vi "nearCamReConnect.vi"(2 "error in":errorcluster, 3 "Session In":T1) -> (0 "错误输出":errorcluster, 1 "IMAQdx Session Out":T1)   [LabVIEW 2018]
uses:
  <vilib>/userdefined/High Color/IMAQdx.ctl
  <vilib>/vision/driver/NI_Vision_Acquisition_Software.lvlib
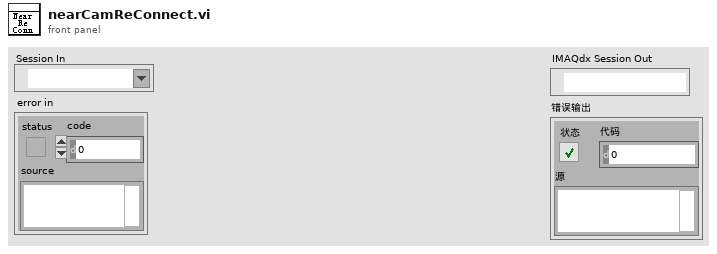
[diagram p1: front panel]
types:
  T1 = typedef "IMAQdx.ctl" = refnum<k21>
  T2 = typedef "IMAQ Image.ctl" = refnum<image>
  T3 = cluster{"示波器":cluster{"Channel (0:Channel 1)":enum16{"Channel 1", "Channel 2", "Channel 3", "Channel 4"}, "电压范围":dbl, "触发电压":dbl, "时间范围":dbl, " 示波器VISA":refnum<visa-resource-name>, "时间范围 标签":u64, "电压范围 标签":u64, "触发电压 标签":u64, "输入阻抗/Ω":u64}, "光谱仪":cluster{"SpecDataReference":refnum<queue>, "grating center":dbl, "Exposure Time (s)":dbl, "是否进行详细设置":bool, " 开始通信检查":bool, "通信成功？":bool, "波长":dbl}, " 近场相机":cluster{"曝光时间/us":dbl, "模拟增益":i32, "控制套接字":i32, "IP 地址":string, " 采集套接字":i32, "  版本号":i32, "ImageData":T2, "  增益最大":i32, "  增益最小":i32, " 曝光最大":i32, " 曝光最小":i32, " 帧速":i32, " 同步切换":i32, "  曝光缩放":i32, "Camera Source":refnum<k21>, "近场X范围":dbl, "近场Y范围":dbl, "单个像元大小/um":dbl, "相机距离原点位置":dbl[], "是否测量发散角":bool, "光束类型(发散T)":bool, "聚焦透镜焦距mm":dbl}, " 偏振仪":cluster{"电压范围":u64, "触发电压":u64, "时间范围":u64, "波长范围":enum16{"可见光 400-700nm", "近红外 700-1100nm"}, "可见光偏振测量仪VISA":refnum<visa-resource-name>, "近红外偏振测量仪VISA":refnum<visa-resource-name>}, " 功率计":cluster{"通道":enum16{"Channel 1", "Channel 2"}, "工作波长":u32, "单位":u64, "时间范围":u64, "IP地址":string, "端口":u32, "是否需要散射片":bool}, "能量计":cluster{"通道":enum16{"Channel 1", "Channel 2"}, "工作波长":u32, "单位":u64, "时间范围":u64, "IP地址":string, "端口":u32, "能量计量程":enum16{"200uJ", "20uJ", "2uJ", "200nJ"}}, "电机":cluster{"Channel (0:Channel 1)":enum16{"Channel 1", "Channel 2", "Channel 3", "Channel 4"}, "电压范围":u64, "触发电压":u64, "时间范围":u64}, " 远场相机":cluster{"曝光时间":i32, "模拟增益":i32, "控制套接字":i32, "IP 地址":string, " 采集套接字":i32, "  版本号":i32, "ImageData":T2, "  增益最大":i32, "  增益最小":i32, " 曝光最大":i32, " 曝光最小":i32, " 帧速":i32, " 同步切换":i32, "  曝光缩放":i32, "ImageData B":T2, "是否远场测量":bool}}
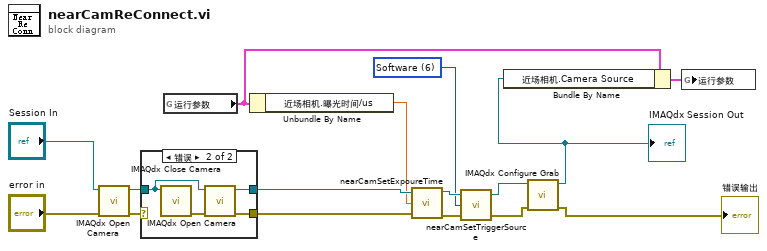
[diagram p0: block diagram]
diagram:
  w8 = u16 6 items=["Freerun"=0, "Line1"=1, "Line2"=2, "FixedRate"=5, "Software"=6] ("Sourece")
  n1 = call <vilib>:"IMAQdx Open Camera.vi"("error in"="error in", "Session In"="Session In") -> ("error out"=w15:errorcluster, "Session Out"=w16:T1)  [unwired: 8 in]
  n2 = case shown="错误" w15 {
    selector: w15 -> [w17 _]
    tunnel: w16 -> [w18 w21]
    tunnel: [w18 w20] -> w13
    tunnel: [w17 w19] -> w10
    frame No Error {
    }
    frame Error {
      n3 = call <vilib>:"IMAQdx Close Camera.vi"("Session In"=w21) -> ("error out"=w22:errorcluster)  [unwired: 10 in]
      n4 = call <vilib>:"IMAQdx Open Camera.vi"("error in"=w22, "Session In"=w21) -> ("error out"=w19:errorcluster, "Session Out"=w20:T1)  [unwired: 8 in]
    }
  }
  n5 = global read "参数.vi" "运行参数"() -> (w6:T3)
  n6 = Unbundle By Name(w6) -> ("近场相机.曝光时间/us"=w9:dbl)
  n7 = call "nearCamSetExpoureTime.vi"("错误输入（无错误）"=w10, "Time/us"=w9, "IMAQdx Session"=w13) -> ("错误输出"=w11:errorcluster, "IMAQdx Session Out"=w12:T1)  [unwired: 1 in, 3 out]
  n8 = call "nearCamSetTriggerSource.vi"("错误输入（无错误）"=w11, "Sourece"=w8, "IMAQdx Session"=w12) -> ("错误输出"=w3:errorcluster, "IMAQdx Session Out"=w4:T1)  [unwired: 1 in]
  n9 = call <vilib>:"IMAQdx Configure Grab.vi"("error in"=w3, "Session In"=w4) -> ("error out"=→"错误输出":errorcluster, "Session Out"=w2:T1)  [unwired: 8 in]
  "IMAQdx Session Out" <- w2
  n10 = Bundle By Name(cluster=w6, "近场相机.Camera Source"=w2) -> (w5:T3)
  n11 = global write "参数.vi" "运行参数"(w5) -> ()
